vi "功能计算_何 截取位移右.vi"(0 "位移数组":dbl[](array[numeric]), 2 "拉压力数组":dbl[](array[numeric]), 3 "半行程":dbl, 5 "截取百分比":dbl) -> (14 "峰值扭矩":dbl format="%#.2f", 16 "最小扭矩":dbl, 17 "平均扭矩":dbl format="%#.2f", 19 "扭差":dbl format="%#.2f")   [LabVIEW 2013]
panel:
  out "第一个子数组":dbl[](array[numeric])
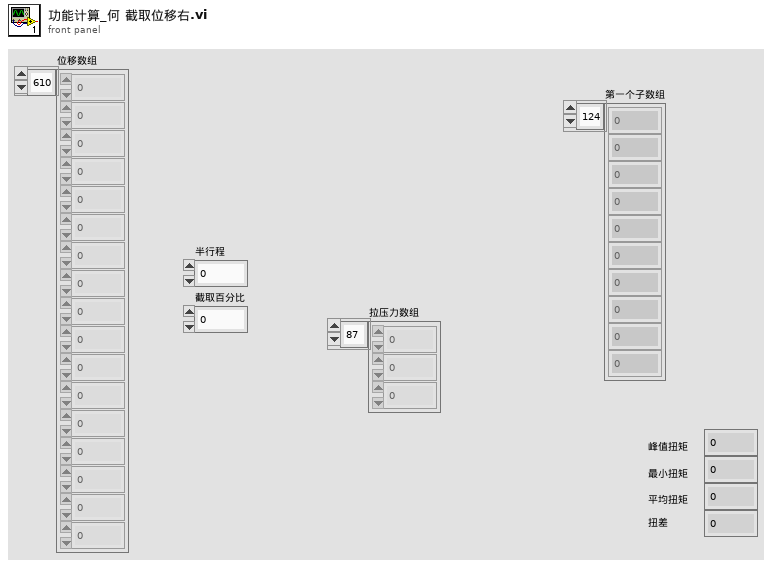
[diagram p1: front panel]
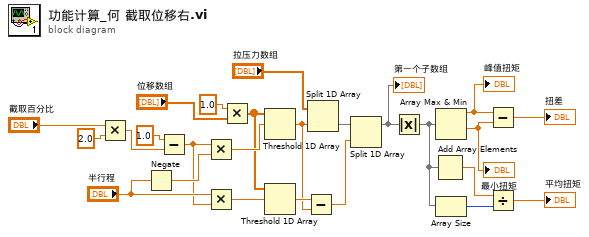
[diagram p0: block diagram]
diagram:
  n1 = Multiply(x="截取百分比", y=2.0) -> (x*y=w2:dbl)
  n2 = Negate(x="半行程") -> (-x=w9:dbl)
  n3 = Subtract(x=1.0, y=w2) -> (x-y=w8:dbl)
  n4 = Multiply(x=w8, y=w9) -> (x*y=w13:dbl)
  n5 = Multiply(x="半行程", y=w8) -> (x*y=w10:dbl)
  n6 = Multiply(x=1.0, y="位移数组") -> (x*y=w12:dbl[])
  n7 = Threshold 1D Array(2:w13, 3:w12) -> (0:w4:dbl)  [unwired: 1 in]
  n8 = Threshold 1D Array(2:w10, 3:w12) -> (0:w5:dbl)  [unwired: 1 in]
  n9 = Subtract(x=w5, y=w4) -> (x-y=w17:dbl)
  n10 = Split 1D Array(array="拉压力数组", index=w4) -> (second subarray=w18:dbl[])  [unwired: 1 out]
  n11 = Split 1D Array(array=w18, index=w17) -> (first subarray=w22:dbl[])  [unwired: 1 out]
  "第一个子数组" <- w22
  n12 = Absolute Value(x=w22) -> (abs(x)=w24:dbl[])
  n13 = Add Array Elements(numeric array=w24) -> (sum=w25:dbl)
  n14 = Array Max & Min(array=w24) -> (max value=w21:dbl, min value=w3:dbl)  [unwired: 2 out]
  "峰值扭矩" <- w21
  "最小扭矩" <- w3
  n15 = Array Size(array=w24) -> (size(s)=w23:i32)
  n16 = Subtract(x=w21, y=w3) -> (x-y=→"扭差":dbl)
  n17 = Divide(x=w25, y=w23) -> (x/y=→"平均扭矩":dbl)
